vi "PH_ImageOperator.ProcPeriodic.vi"(0 "i ref in":refnum<vi>, 3 "ms timeout (100)":i32=100, 5 "error in (no error)":errorcluster) -> (14 "i ref out":refnum<vi>, 17 "timed out":bool, 19 "error out":errorcluster)   [LabVIEW 2014, in "PH_ImageOperator.lvlib"]
doc: "This method serves to periodically do things like reading values from the HW. Methods that should be executed periodically should be called from THIS methode. Add code here."
uses:
  PH_ImageOperator.lvlib
  PH_Basics/PH_Img_BaseClass/PH_Img_BaseClass.lvlib
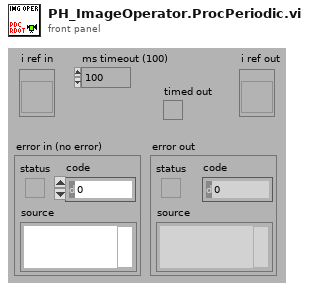
[diagram p1: front panel]
types:
  T1 = typedef "IMAQ Image.ctl" = refnum<image>
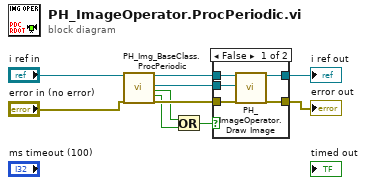
[diagram p0: block diagram]
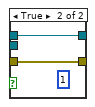
[diagram p2: hidden frame]
diagram:
  n1 = call "PH_Img_BaseClass.ProcPeriodic.vi"("i ref in"="i ref in", "error in (no error)"="error in (no error)") -> ("i ref out"=w7:refnum<vi>, "Cam Image"=w4:T1, "timed out?"=w3:bool, "Error while unflatten data?"=w2:bool, "error out"=w5:errorcluster)  [unwired: 13 in]
  n2 = Or(x=w3, y=w2) -> (x .or. y?=w1:bool)
  n3 = case shown="False" w1 {
    tunnel: w7 -> [w15 w17]
    tunnel: [w12 w17] -> w9
    tunnel: w5 -> [w14 w16]
    tunnel: [w13 w16] -> w6
    tunnel: w4 -> [w11 _]
    frame False {
      n4 = call "PH_ImageOperator.Draw Image.vi"("i ref in"=w15, "Cam Image"=w11, "error in (no error)"=w14) -> ("i ref out"=w12:refnum<vi>, "error out"=w13:errorcluster)  [unwired: 15 in]
    }
    frame True {
      (unwired) 1
    }
  }
  "error out" <- w6
  "i ref out" <- w9
